vi "AI_Read.vi"(8 "error in (no error)":errorcluster, 9 "Stop AI":bool, 11 "reference in":refnum<class "AI.lvclass">) -> (0 "error out":errorcluster, 3 "reference out":refnum<class "AI.lvclass">)   [LabVIEW 2017, in "AI.lvclass"]
uses:
  AI.lvclass
panel:
  # "This VI is called Asynchronously and will have one instance in memory\nfor each asynchronous call."
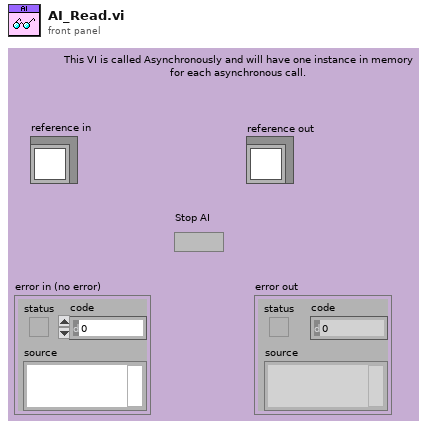
[diagram p1: front panel]
types:
  T1 = typedef "AI.lvclass/ObjectAttributes.ctl" = cluster{"AI Task":refnum<k21>, "AI On/Off Status":bool, "AI Sampling Rate (Samples/Seconds)":u32, "Number of AI Samples Per Channel":i32, "AI Voltage Range":u8, "AI Readings":dbl[][], "Number of AI Modules":i32, "Number of Total AI Channels":i32, "AI Module Names (NI-Max Name)":string[], "Number of Channels Per AI  Module":i32[], "AI VI Reference":refnum<vi>}
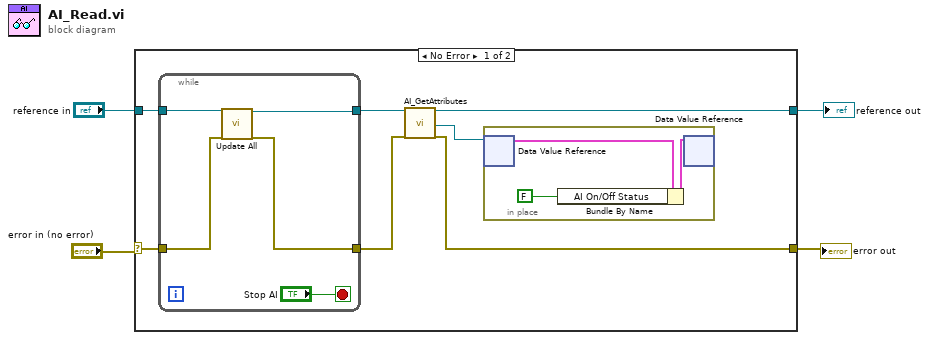
[diagram p0: block diagram]
diagram:
  n1 = case shown="No Error" "error in (no error)" {
    selector: "error in (no error)" -> [w11 w20]
    tunnel: [w5 w20] -> w3
    tunnel: "reference in" -> [w10 w21]
    tunnel: [w8 w21] -> w2
    frame No Error {
      n2 = while {
        tunnel: [w14] -> w6
        tunnel: w11 -> [w15]
        tunnel: w10 -> [w13]
        tunnel: [w12] -> w9
        stop <- "Stop AI" stop-if-true
        n3 = call-dynamic "Update All.vi"("reference in"=w13, "error in (no error)"=w15) -> ("reference out"=w12:refnum<class "AI.lvclass">, "error out"=w14:errorcluster)  [unwired: 16 in]
      }
      n4 = call "AI_GetAttributes.vi"("reference in"=w9, "error in (no error)"=w6) -> ("reference out"=w8:refnum<class "AI.lvclass">, "DataRef"=w7:refnum<data-value>, "error out"=w5:errorcluster)  [unwired: 14 in, 1 out]
      n5 = in-place {
        n6 = in-place-dvr #1(w7) -> (w19:T1)  [unwired: 1 out]
        n7 = Bundle By Name(cluster=w19, "AI On/Off Status"=FALSE ("DO On/Off Status")) -> (w18:T1)
        n8 = in-place-dvr #1(w18) -> ()  [unwired: 2 out]
      }
    }
    frame Error {
    }
  }
  "error out" <- w3
  "reference out" <- w2
